vi "Write Variable (one-row).vi"(6 "Time Stamp":timestamp, 8 "error in (no error)":errorcluster, 9 "Data":variant, 10 "Paths":variant, 11 "Data.PG in":refnum<class "LV-Data.PGSQL.lvclass">) -> (0 "error out":errorcluster, 1 "Wrote to DB?":bool, 2 "Paths out":string, 3 "Data.PG out":refnum<class "LV-Data.PGSQL.lvclass">)   [LabVIEW 2019, in "LV-Data.PGSQL.lvclass"]
uses:
  LV-Data.PGSQL.lvclass
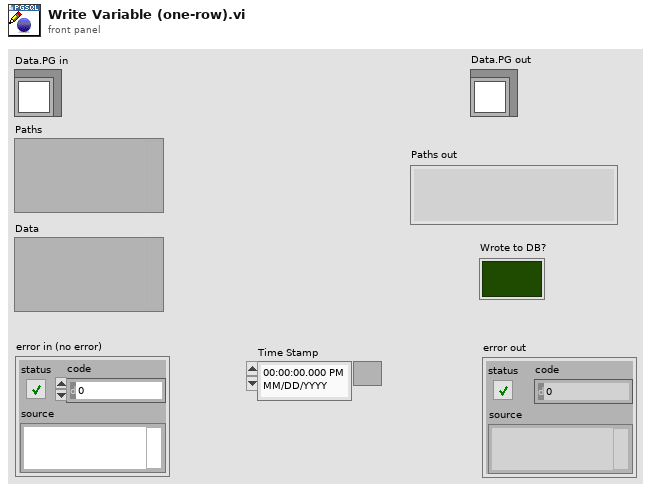
[diagram p1: front panel]
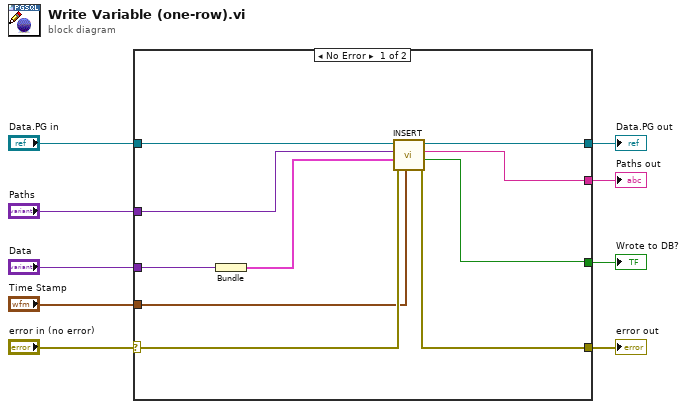
[diagram p0: block diagram]
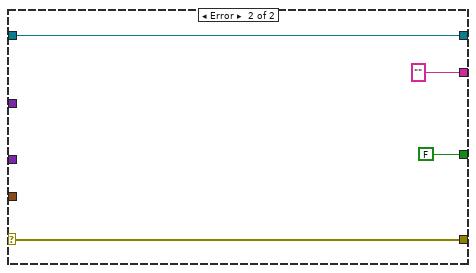
[diagram p2: hidden frame]
diagram:
  n1 = case shown="No Error" "error in (no error)" {
    selector: "error in (no error)" -> [w14 w23]
    tunnel: "Data.PG in" -> [w19 w22]
    tunnel: [w11 FALSE ("Wrote to DB?")] -> w8
    tunnel: "Paths" -> [w18 _]
    tunnel: "Data" -> [w17 _]
    tunnel: [w16 w22] -> w5
    tunnel: [w13 w23] -> w3
    tunnel: "Time Stamp" -> [w12 _]
    tunnel: [w10 "" ("Paths out")] -> w1
    frame No Error {
      n2 = Bundle("Data"=w17) -> (w15:cluster{"Data":variant})  [unwired: 1 in]
      n3 = call "INSERT.vi"("Time Stamp"=w12, "error in"=w14, "Data"=w15, "Path(s)"=w18, "Data.PG in"=w19) -> ("error out"=w13:errorcluster, "Wrote to DB?"=w11:bool, "Paths out"=w10:string, "Data.PG out"=w16:refnum<class "LV-Data.PGSQL.lvclass">)  [unwired: 3 in]
    }
    frame Error {
    }
  }
  "Wrote to DB?" <- w8
  "Data.PG out" <- w5
  "error out" <- w3
  "Paths out" <- w1
